vi "ADV Compute.vi"(8 "error in":errorcluster, 10 "ADV String":string, 11 "Water Tunnel Results in":refnum<class "Water Tunnel Results.lvclass">) -> (0 "error out":errorcluster, 1 "ADV":waveform(dbl)[](array[waveform]), 2 "ADV Rav":waveform(dbl)[](array[waveform]), 3 "Water Tunnel Results out":refnum<class "Water Tunnel Results.lvclass">)   [LabVIEW 2019, in "Results.lvlib" / "Water Tunnel Results.lvclass"]
uses:
  Water Tunnel Results.lvclass
  Water Tunnel Results.lvclass/Water Tunnel Results.ctl
panel:
  out "Array":waveform(dbl)[](array[waveform])
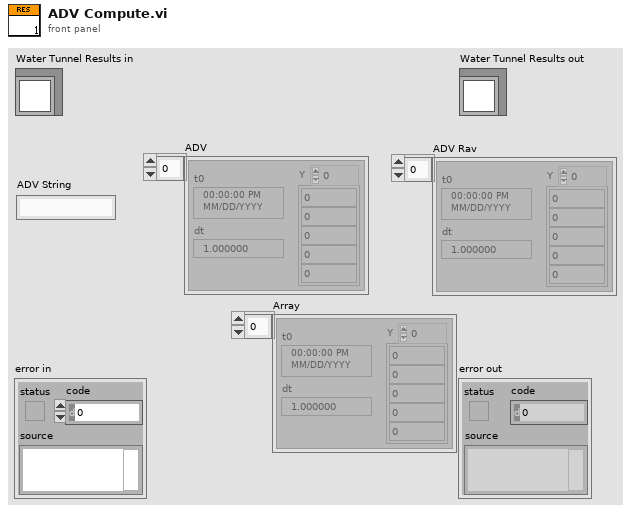
[diagram p1: front panel]
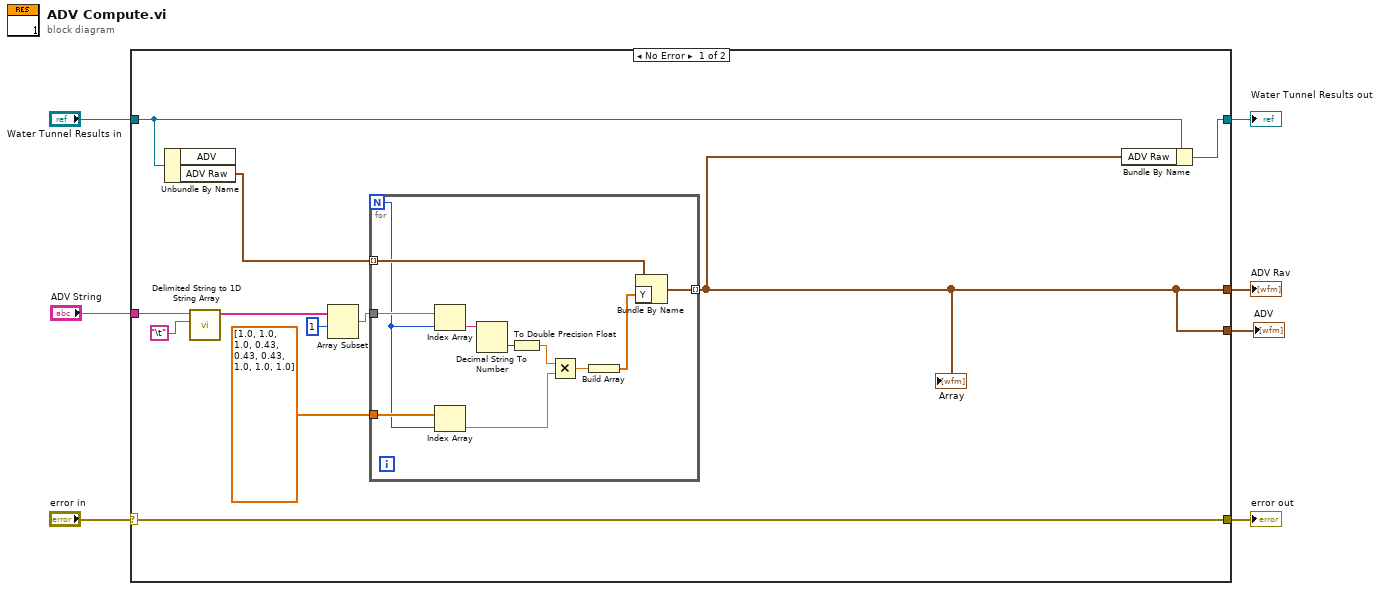
[diagram p0: block diagram]
diagram:
  n1 = case shown="No Error" "error in" {
    selector: "error in" -> [w18 w31]
    tunnel: [w18 w31] -> w6
    tunnel: [w17 w30] -> w4
    tunnel: "Water Tunnel Results in" -> [w16 w30]
    tunnel: "ADV String" -> [w15 _]
    tunnel: [w11 _] -> w2
    tunnel: [w11 _] -> w1
    frame No Error {
      n2 = Unbundle By Name(w16) -> ("ADV Raw"=w13:waveform(dbl)[])  [unwired: 1 out]
      n3 = call <vilib>:"Delimited String to 1D String Array.vi"("delimiter"="\t", "delimited string"=w15) -> ("string array"=w10:string[])  [unwired: 9 in]
      n4 = Array Subset(array=w10, index=1) -> (w8:string[])  [unwired: 1 in]
      n5 = for {
        N -> [w25]
        tunnel: w13 -> [w29] mode=indexing
        tunnel: w8 -> [w28]
        tunnel: dbl[] [1.0, 1.0, 1.0, 0.43, 0.43, 0.43, 1.0, 1.0, 1.0] -> [w26]
        tunnel: [w19] -> w11 mode=indexing
        n6 = Index Array(array=w28, index=w25) -> (element=w27:string)
        n7 = Index Array(array=w26, index=w25) -> (element=w24:dbl)
        n8 = Decimal String To Number(string=w27) -> (number=w23:i32)  [unwired: 2 in, 1 out]
        n9 = To Double Precision Float(number=w23) -> (double precision float=w22:dbl)
        n10 = Multiply(x=w22, y=w24) -> (x*y=w21:dbl)
        n11 = Build Array(w21) -> (w20:dbl[])
        n12 = Bundle By Name(cluster=w29, "Y"=w20) -> (w19:waveform(dbl))
      }
      "Array" <- w11
      n13 = Bundle By Name(cluster=w16, "ADV Raw"=w11) -> (w17:refnum<class "Water Tunnel Results.lvclass">)
    }
    frame Error {
    }
  }
  "error out" <- w6
  "Water Tunnel Results out" <- w4
  "ADV" <- w1
  "ADV Rav" <- w2
